vi "Autonomous Independent.vi"() -> ()   [LabVIEW 2015]
doc: "This VI is called when autonomous begins, and will automatically be terminated when autonomous ends. You can carry out timed or sensor driven robot movement independently without needing to return to the caller."
uses:
  <vilib>/Rock Robotics/WPI/Utilities/WPI_GetSetVariantRefNum.vi
  <vilib>/Rock Robotics/Network Tables/NT Read String.vi
  <vilib>/Rock Robotics/Network Tables/NT Write Numeric Array.vi
  <vilib>/Rock Robotics/Network Tables/NT Write Number.vi
  <vilib>/addons/control/pid/pid.llb/PID (DBL).vi
  Robot Global Data.vi
  <vilib>/Rock Robotics/Network Tables/NT Read Number.vi
  <vilib>/addons/control/pid/NI_PID_pid.lvlib
  navX Library v2/navX Library v2.lvlib
panel:
  in  "Aiming Gains":T1={"proportional gain (Kc)"=1.0, "integral time (Ti, min)"=0.01, "derivative time (Td, min)"=0.0} {"derivative time (Td, min)" format="%.3f"; "integral time (Ti, min)" format="%.3f"; "proportional gain (Kc)" format="%.3f"}
  out "Yaw":dbl(graph)
  in  "Target Angle":dbl=30.0
  out "E1 Rate":dbl
  out "E2 Rate":dbl
  out "Yaw Display":dbl
  in  "Single Turn Gains":T1={"proportional gain (Kc)"=0.12, "integral time (Ti, min)"=0.0, "derivative time (Td, min)"=0.0} {"derivative time (Td, min)" format="%.3f"; "integral time (Ti, min)" format="%.3f"; "proportional gain (Kc)" format="%.3f"}
  in  "Yaw":T1={"proportional gain (Kc)"=0.2, "integral time (Ti, min)"=0.0, "derivative time (Td, min)"=0.0} {"derivative time (Td, min)" format="%.3f"; "integral time (Ti, min)" format="%.3f"; "proportional gain (Kc)" format="%.3f"}
  out "Right Motor Speed":dbl(graph)
  out "Left Motor Speed":dbl(graph)
  out "Right Motor":dbl(graph)
  out "Left Motor":dbl(graph)
  in  "Distance":dbl=120.0
  in  "Speed Gains":T1={"proportional gain (Kc)"=0.65, "integral time (Ti, min)"=0.001, "derivative time (Td, min)"=0.001} {"derivative time (Td, min)" format="%.3f"; "integral time (Ti, min)" format="%.3f"; "proportional gain (Kc)" format="%.3f"}
  out "E2 Dist":dbl
  out "E1 Dist":dbl
  # "Be sure to right-click and choose Data Operations>>Make Current Value default if you want to save the array values with the VI"
  # "Encoder Distance Traveled"
  # "Speed we are assigning the motors and Encoder Rate"
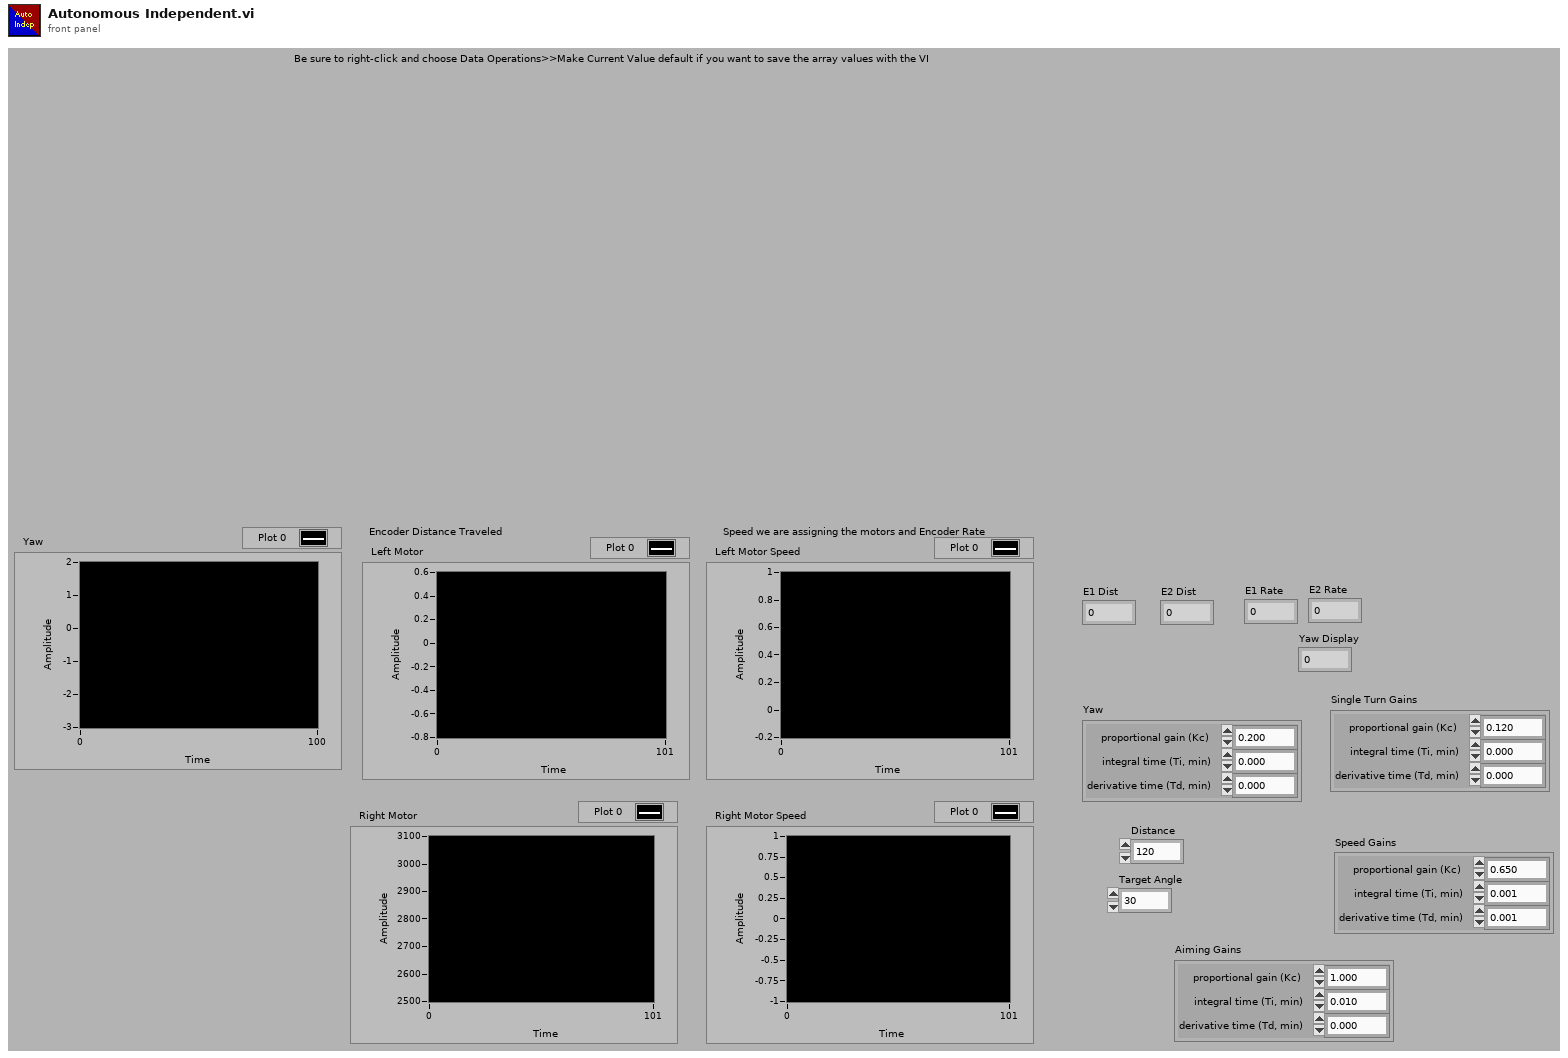
[diagram p1: front panel]
types:
  T1 = cluster{"proportional gain (Kc)":dbl, "integral time (Ti, min)":dbl, "derivative time (Td, min)":dbl}
  T2 = typedef "WPI_JoystickDevRef.ctl" = cluster{"Device":T3}
  T3 = typedef "WPI_JoystickDeviceEnum.ctl" = enum16{"USB 0", "USB 1", "USB 2", "USB 3", "USB 4", "USB 5"}
  T4 = typedef "navX Library v2.lvlib/Z900_navX_DeviceTypeDef.ctl" = cluster{"Interface":cluster{"Protocol":T5, "Update Rate (4Hz-60Hz)":u8, "navX Open TypeDef":variant}, "Notify Packet":refnum<notifier>, "Loop VI Refnum":refnum<vi>, "Ready to Close Occurrence Refnum":refnum<k4>}
  T5 = typedef "navX Library v2.lvlib/Z900_navX_ProtocolTypeDef.ctl" = enum16{"SERIAL", "I2C", "SPI"}
  T6 = typedef "WPI_EncoderDevRef.ctl" = cluster{"DevStatus":errorcluster, "EncoderIndex":T7, "CounterIndex":T8, "DistancePerCount":dbl, "Decoding Type":T9}
  T7 = typedef "FPGA_EncoderIdx.ctl" = enum8{"Enc 0", "Enc 1", "Enc 2", "Enc 3", "Enc 4", "Enc 5", "Enc 6", "Enc 7", "Invalid"}
  T8 = typedef "FPGA_CounterCtrSystemIndex.ctl" = enum8{"Ctr 0", "Ctr 1", "Ctr 2", "Ctr 3", "Ctr 4", "Ctr 5", "Ctr 6", "Ctr 7", "Invalid"}
  T9 = typedef "WPI_EncoderType.ctl" = enum16{"1x", "2x", "4x"}
  T10 = cluster{"Yaw":dbl, "Roll":dbl, "Pitch":dbl, "Heading":dbl, "Fused Heading":dbl}
  T11 = typedef "WPI_RobotDriveDevRef.ctl" = cluster{"DevStatus":errorcluster, "Motors[]":T12[], "Square Inputs":bool, "Max Output":dbl}
  T12 = typedef "WPI_MotorControlDeviceRef.ctl" = cluster{"DeviceStatus":errorcluster, "Type":T13, "PWM":cluster{"PWM Channel":T14, "DeadBand":T15}, "CAN":cluster{"Device Number":u8, "Control Mode":T16, "Semaphore":T17, "Max Vout":dbl, "TalonSRX Control Mode":T18}, "Invert":bool}
  T13 = typedef "WPI_MotorControlType.ctl" = enum16{"PWM", "CAN", "CANTalonSRX"}
  T14 = typedef "FPGA_DIOPWMChannel.ctl" = enum8{"PWM 0", "PWM 1", "PWM 2", "PWM 3", "PWM 4", "PWM 5", "PWM 6", "PWM 7", "PWM 8", "PWM 9", "PWM MXP 0", "PWM MXP 1", "PWM MXP 2", "PWM MXP 3", "PWM MXP 4", "PWM MXP 5", "PWM MXP 6", "PWM MXP 7", "PWM MXP 8", "PWM MXP 9", "Invalid"}
  T15 = typedef "WPI_PWMDeadband.ctl" = cluster{"Name":string, "maxPositivePwm":i32, "minPositivePwm":i32, "centerPwm":i32, "maxNegativePwm":i32, "minNegativePwm":i32, "angularRange":u16}
  T16 = typedef "WPI_CANJaguar_ControlMode.ctl" = enum8{"Percent VBus", "Current", "Speed", "Position", "Voltage"}
  T17 = typedef "Semaphore RefNum" = refnum<k1>
  T18 = typedef "WPI_CANTalonSRX_APIControlMode.ctl" = enum8{"Percent VBus", "Speed", "Position", "Slave", "Unchanged / Invalid", "Voltage Compensation", "Current", "Motion Profile"}
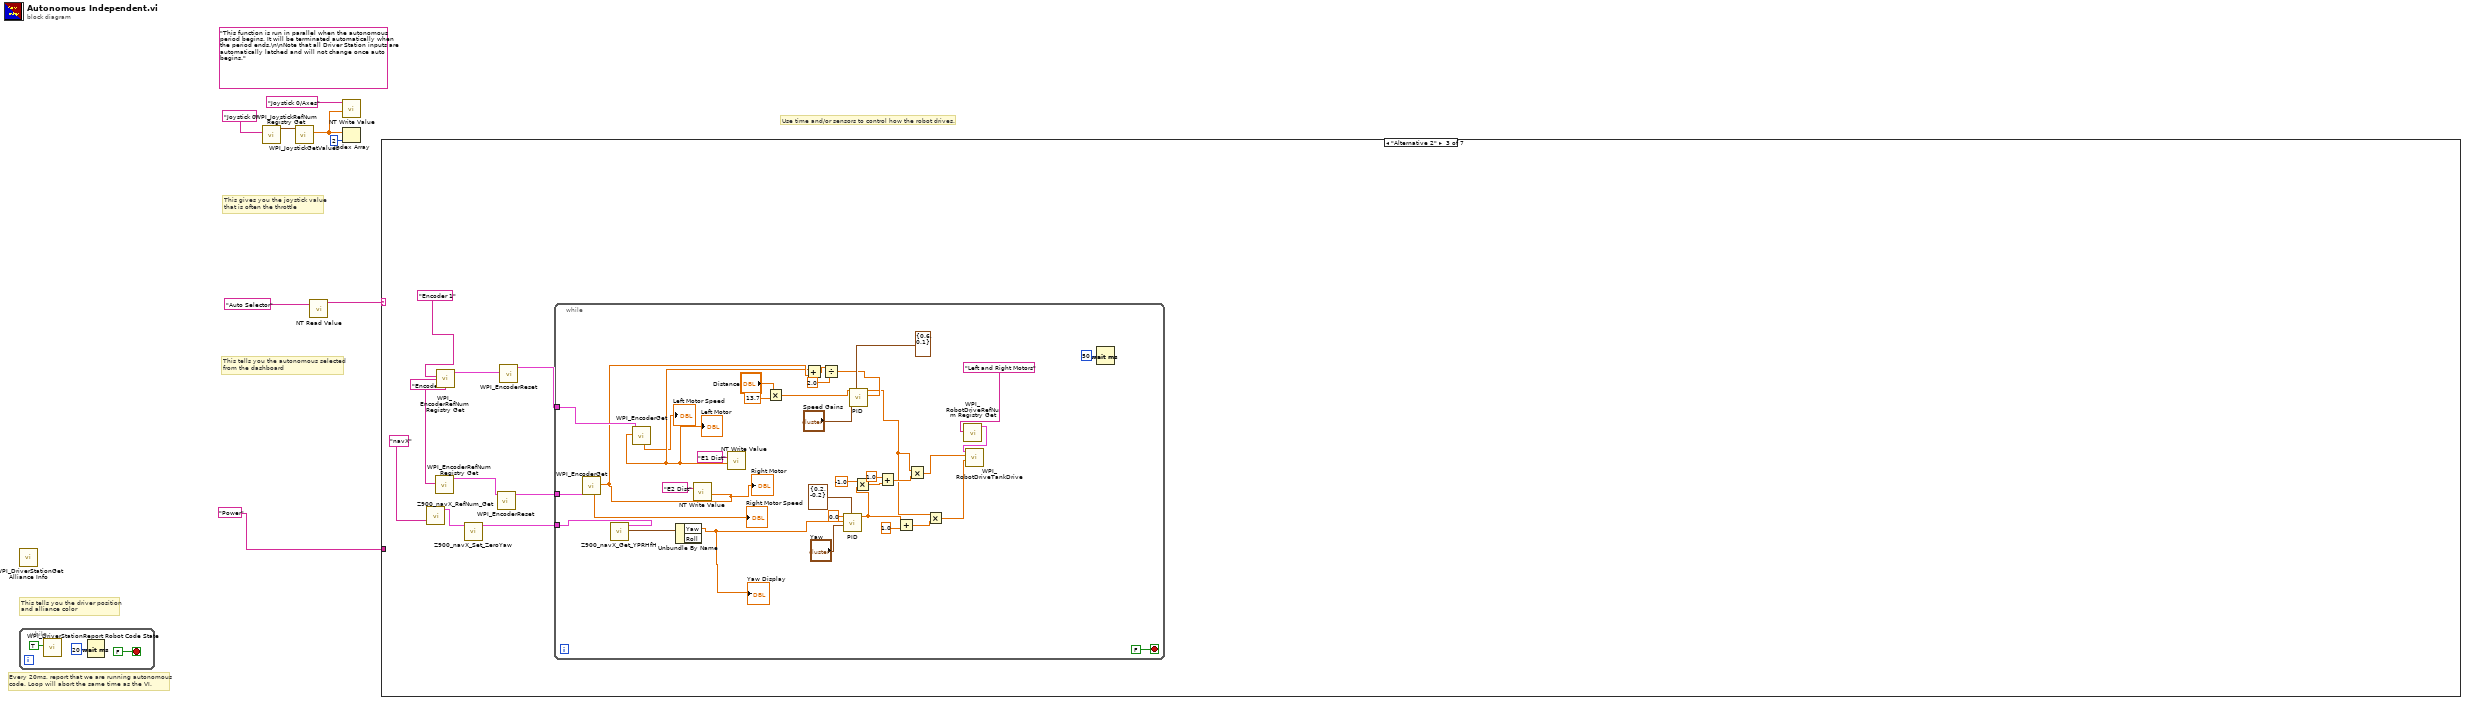
[diagram p0: block diagram]
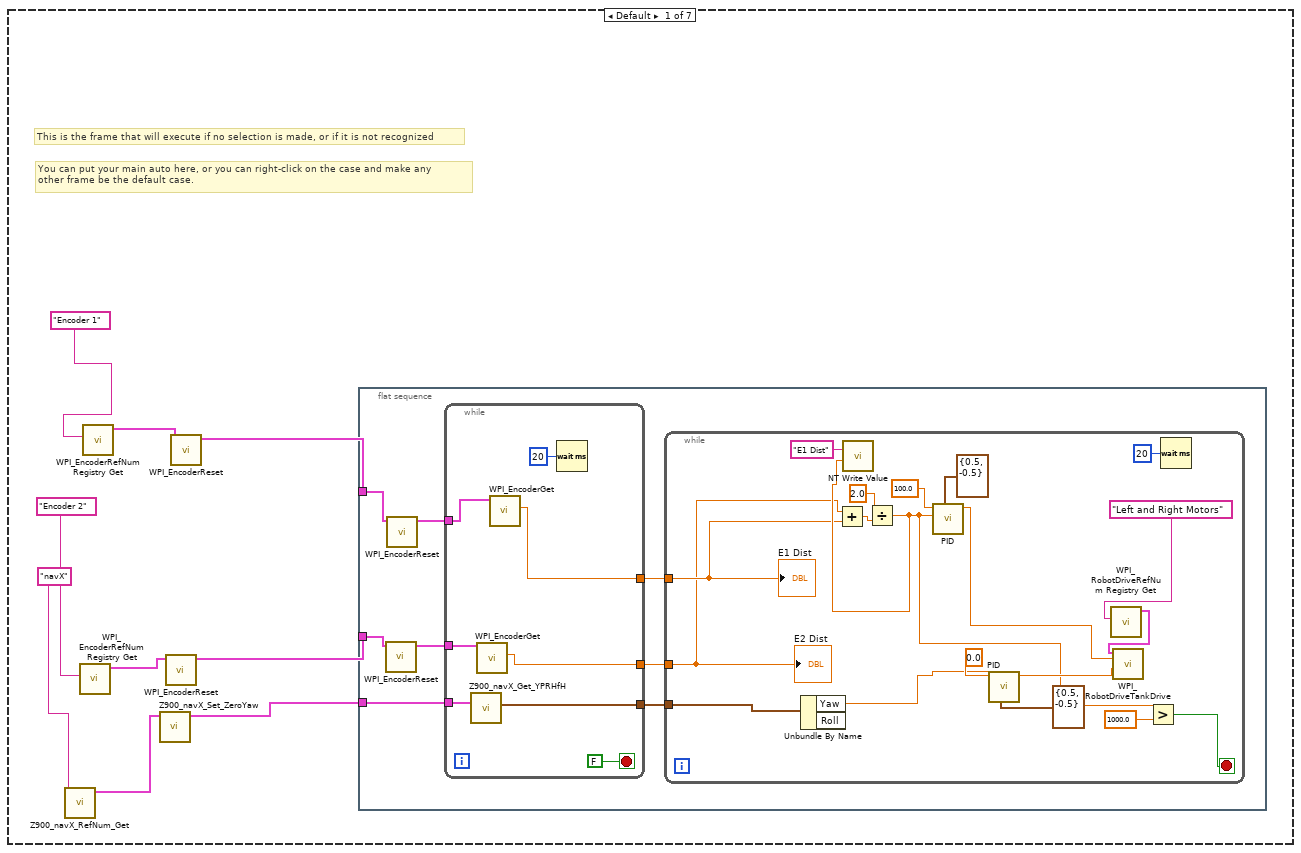
[diagram p2: hidden frame]
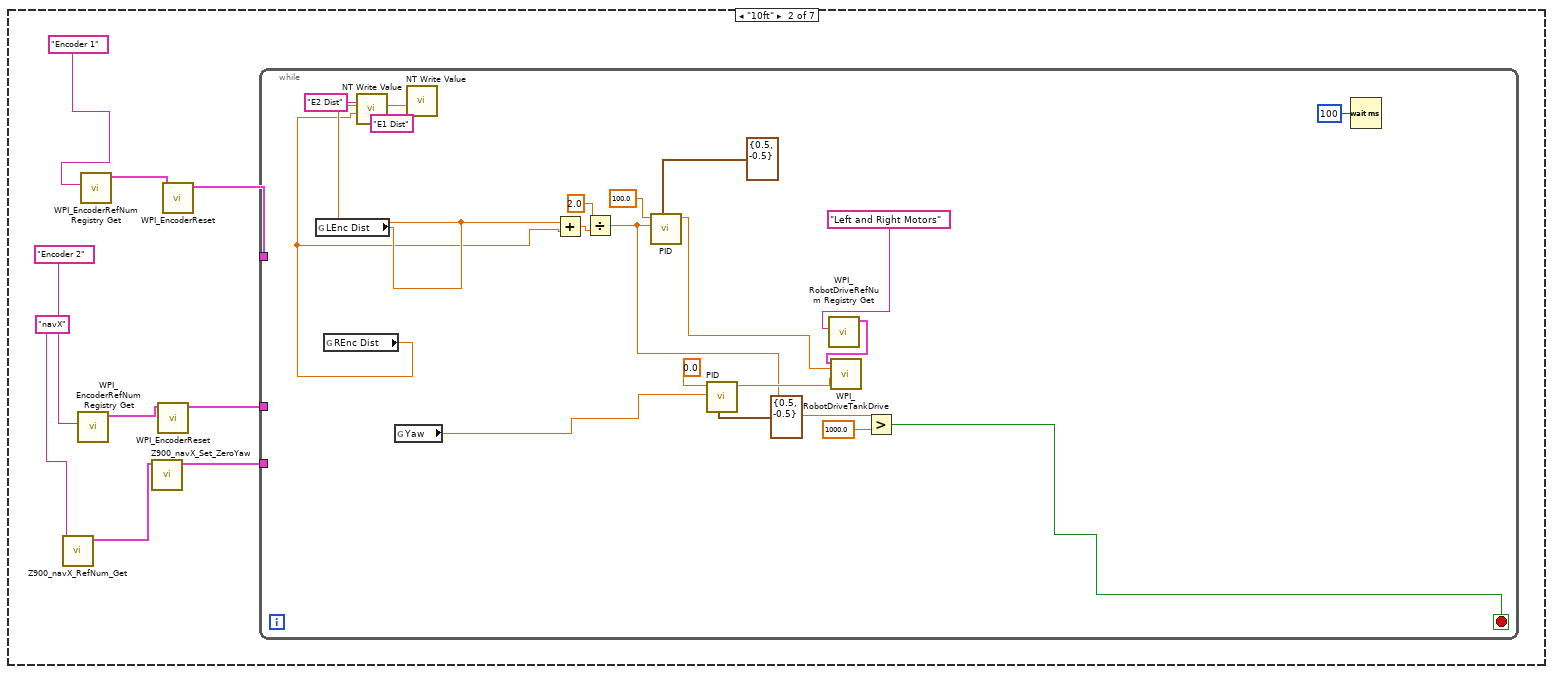
[diagram p3: hidden frame]
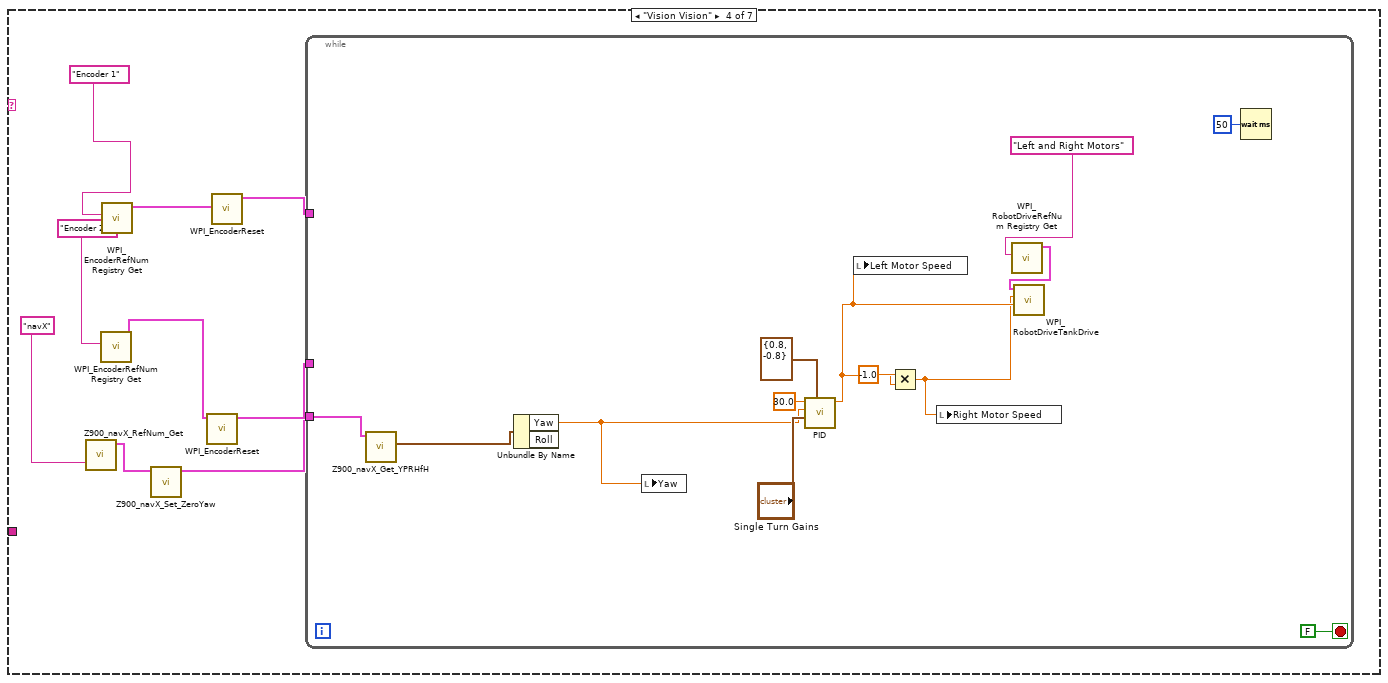
[diagram p4: hidden frame]
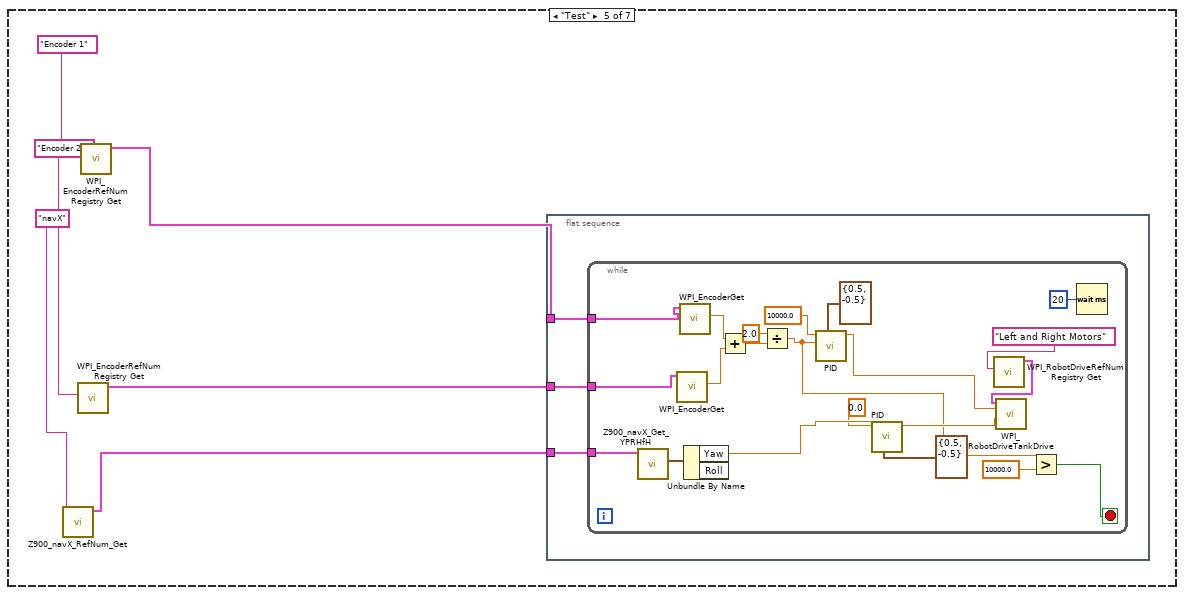
[diagram p5: hidden frame]
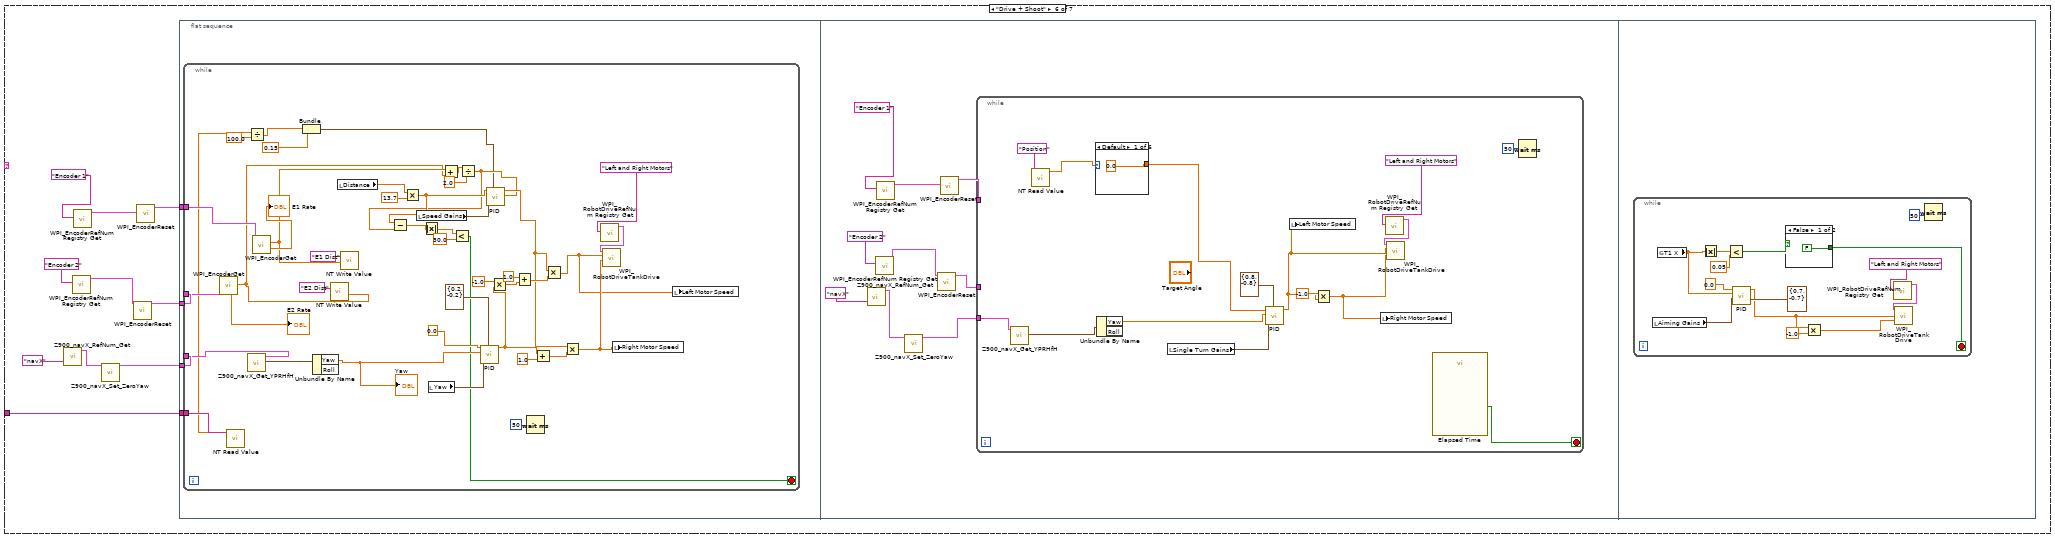
[diagram p6: hidden frame]
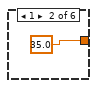
[diagram p7: hidden frame]
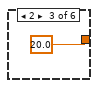
[diagram p8: hidden frame]
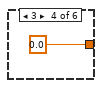
[diagram p9: hidden frame]
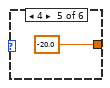
[diagram p10: hidden frame]
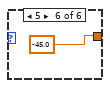
[diagram p11: hidden frame]
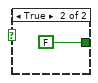
[diagram p12: hidden frame]
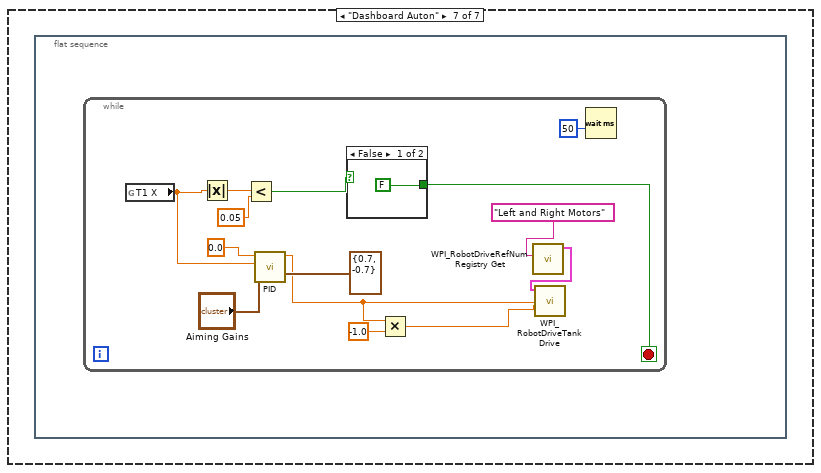
[diagram p13: hidden frame]
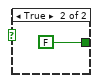
[diagram p14: hidden frame]
diagram:
  (unwired) "This function is run in parallel when the autonomous period begins. It will be terminated automatically when the period ends.\n\nNote that all Driver Station inputs are automatically latched and will not change once auto begins."
  # "This tells you the autonomous selected\nfrom the dashboard"
  # "Every 20ms, report that we are running autonomous\ncode. Loop will abort the same time as the VI."
  # "This gives you the joystick value\nthat is often the throttle"
  # "Use time and/or sensors to control how the robot drives."
  # "This tells you the driver position\nand alliance color"
  n1 = while {
    stop <- FALSE stop-if-true
    n2 = call <vilib>:"WPI_DriverStationReport Robot Code State.vi"("Autonomous"=TRUE) -> ()  [unwired: 10 in, 1 out]
    n3 = Wait (ms)(milliseconds to wait=u32 20) -> ()  [unwired: 1 out]
  }
  n4 = call <vilib>:"WPI_DriverStationGet Alliance Info.vi"() -> ()  [unwired: 12 out]
  n5 = call <vilib>:"WPI_JoystickRefNum Registry Get.vi"("refnum name"="Joystick 0") -> ("JoystickDevRef"=w7:T2)  [unwired: 1 in, 9 out]
  n6 = call <vilib>:"WPI_JoystickGetValues.vi"("JoystickDevRef"=w7) -> ("Axes"=w3:dbl[])  [unwired: 6 in, 4 out]
  n7 = call-poly <vilib>:"NT Read Value.vi"("Name"="Auto Selector") -> ("String"=w4:string)  [unwired: 9 in, 1 out]
  n8 = call-poly <vilib>:"NT Write Value.vi"("Numeric Array"=w3, "Name"="Joystick 0/Axes") -> ()  [unwired: 9 in, 1 out]
  n9 = Index Array(array=w3, index=2) -> ()  [unwired: 1 out]
  n10 = case shown="\"Alternative 2\"" w4 {
    tunnel: "Power" ("Name") -> [_ _ _ _ _ w181 _]
    frame Default {
      # "You can put your main auto here, or you can right-click on the case and make any\nother frame be the default case."
      # "This is the frame that will execute if no selection is made, or if it is not recognized"
      n11 = call "Z900_navX_RefNum_Get.vi"("refnum name"="navX") -> ("navX Device"=w14:T4)  [unwired: 9 in, 1 out]
      n12 = call <vilib>:"WPI_EncoderRefNum Registry Get.vi"("refnum name"="Encoder 2") -> ("EncoderDevRef"=w16:T6)  [unwired: 9 in, 1 out]
      n13 = call <vilib>:"WPI_EncoderRefNum Registry Get.vi"("refnum name"="Encoder 1") -> ("EncoderDevRef"=w18:T6)  [unwired: 9 in, 1 out]
      n14 = call "Z900_navX_Set_ZeroYaw.vi"("navX Device"=w14) -> ("navX Device"=w13:T4)  [unwired: 9 in, 1 out]
      n15 = call <vilib>:"WPI_EncoderReset.vi"("EncoderDevRef"=w16) -> ("EncoderDevRef"=w15:T6)  [unwired: 9 in, 1 out]
      n16 = call <vilib>:"WPI_EncoderReset.vi"("EncoderDevRef"=w18) -> ("EncoderDevRef"=w17:T6)  [unwired: 9 in, 1 out]
      n17 = flat-sequence {
        tunnel: w17 -> [w28]
        tunnel: w15 -> [w27]
        tunnel: w13 -> [w26]
        frame #0 {
          n18 = call <vilib>:"WPI_EncoderReset.vi"("EncoderDevRef"=w27) -> ("EncoderDevRef"=w25:T6)  [unwired: 9 in, 1 out]
          n19 = call <vilib>:"WPI_EncoderReset.vi"("EncoderDevRef"=w28) -> ("EncoderDevRef"=w24:T6)  [unwired: 9 in, 1 out]
          n20 = while {
            tunnel: w26 -> [w33]
            tunnel: w25 -> [w34]
            tunnel: w24 -> [w35]
            tunnel: [w32] -> w23
            tunnel: [w31] -> w22
            tunnel: [w30] -> w21
            stop <- FALSE stop-if-true
            n21 = call "Z900_navX_Get_YPRHfH.vi"("navX Device"=w33) -> ("YRPHfH"=w32:T10)  [unwired: 7 in, 3 out]
            n22 = call <vilib>:"WPI_EncoderGet.vi"("EncoderDevRef"=w34) -> ("Distance"=w31:dbl)  [unwired: 5 in, 5 out]
            n23 = call <vilib>:"WPI_EncoderGet.vi"("EncoderDevRef"=w35) -> ("Distance"=w30:dbl)  [unwired: 5 in, 5 out]
            n24 = Wait (ms)(milliseconds to wait=u32 20) -> ()  [unwired: 1 out]
          }
          n25 = while {
            tunnel: w23 -> [w40]
            tunnel: w22 -> [w38]
            tunnel: w21 -> [w39]
            stop <- w44 stop-if-true
            n26 = Unbundle By Name(w40) -> ("Yaw"=w41:dbl)  [unwired: 1 out]
            n27 = Add(x=w38, y=w39) -> (x+y=w55:dbl)
            n28 = Divide(x=2.0, y=w55) -> (x/y=w43:dbl)
            n29 = call-poly <vilib>:"NT Write Value.vi"("Numeric"=w43, "Name"="E1 Dist") -> ()  [unwired: 9 in, 1 out]
            n30 = call-poly <vilib>:"PID.vi"("output range"=cluster{"output high":dbl, "output low":dbl} {"output high"=0.5, "output low"=-0.5}, "process variable"=w43, "setpoint"=100.0) -> ("output"=w48:dbl)  [unwired: 7 in, 1 out]
            n31 = call-poly <vilib>:"PID.vi"("output range"=cluster{"output high":dbl, "output low":dbl} {"output high"=0.5, "output low"=-0.5}, "process variable"=w41, "setpoint"=0.0) -> ("output"=w47:dbl)  [unwired: 7 in, 1 out]
            n32 = call <vilib>:"WPI_RobotDriveRefNum Registry Get.vi"("refnum name"="Left and Right Motors") -> ("RobotDriveDevRef"=w50:T11)  [unwired: 9 in, 1 out]
            n33 = call <vilib>:"WPI_RobotDriveTankDrive.vi"("Right axis value"=w47, "Left axis value"=w48, "RobotDriveDevRef"=w50) -> ()  [unwired: 6 in, 3 out]
            n34 = Greater?(x=w43, y=1000.0) -> (0:w44:bool)
            n35 = Wait (ms)(milliseconds to wait=u32 20) -> ()  [unwired: 1 out]
            "E2 Dist" <- w38
            "E1 Dist" <- w39
          }
        }
      }
    }
    frame "10ft" {
      n36 = call "Z900_navX_RefNum_Get.vi"("refnum name"="navX") -> ("navX Device"=w58:T4)  [unwired: 9 in, 1 out]
      n37 = call <vilib>:"WPI_EncoderRefNum Registry Get.vi"("refnum name"="Encoder 2") -> ("EncoderDevRef"=w60:T6)  [unwired: 9 in, 1 out]
      n38 = call <vilib>:"WPI_EncoderRefNum Registry Get.vi"("refnum name"="Encoder 1") -> ("EncoderDevRef"=w62:T6)  [unwired: 9 in, 1 out]
      n39 = call "Z900_navX_Set_ZeroYaw.vi"("navX Device"=w58) -> ("navX Device"=w57:T4)  [unwired: 9 in, 1 out]
      n40 = call <vilib>:"WPI_EncoderReset.vi"("EncoderDevRef"=w60) -> ("EncoderDevRef"=w59:T6)  [unwired: 9 in, 1 out]
      n41 = call <vilib>:"WPI_EncoderReset.vi"("EncoderDevRef"=w62) -> ("EncoderDevRef"=w61:T6)  [unwired: 9 in, 1 out]
      n42 = while {
        tunnel: w61 -> [_]
        tunnel: w59 -> [_]
        tunnel: w57 -> [_]
        stop <- w65 stop-if-true
        n43 = global read "Robot Global Data.vi" "LEnc Dist"() -> (w68:dbl)
        n44 = global read "Robot Global Data.vi" "REnc Dist"() -> (w67:dbl)
        n45 = call-poly <vilib>:"NT Write Value.vi"("Numeric"=w67, "Name"="E2 Dist") -> ()  [unwired: 9 in, 1 out]
        n46 = global read "Robot Global Data.vi" "Yaw"() -> (w66:dbl)
        n47 = call-poly <vilib>:"NT Write Value.vi"("Numeric"=w68, "Name"="E1 Dist") -> ()  [unwired: 9 in, 1 out]
        n48 = Add(x=w68, y=w67) -> (x+y=w82:dbl)
        n49 = Divide(x=2.0, y=w82) -> (x/y=w72:dbl)
        n50 = call-poly <vilib>:"PID.vi"("output range"=cluster{"output high":dbl, "output low":dbl} {"output high"=0.5, "output low"=-0.5}, "process variable"=w72, "setpoint"=100.0) -> ("output"=w76:dbl)  [unwired: 7 in, 1 out]
        n51 = call-poly <vilib>:"PID.vi"("output range"=cluster{"output high":dbl, "output low":dbl} {"output high"=0.5, "output low"=-0.5}, "process variable"=w66, "setpoint"=0.0) -> ("output"=w75:dbl)  [unwired: 7 in, 1 out]
        n52 = call <vilib>:"WPI_RobotDriveRefNum Registry Get.vi"("refnum name"="Left and Right Motors") -> ("RobotDriveDevRef"=w78:T11)  [unwired: 9 in, 1 out]
        n53 = call <vilib>:"WPI_RobotDriveTankDrive.vi"("Right axis value"=w75, "Left axis value"=w76, "RobotDriveDevRef"=w78) -> ()  [unwired: 6 in, 3 out]
        n54 = Greater?(x=w72, y=1000.0) -> (0:w65:bool)
        n55 = Wait (ms)(milliseconds to wait=u32 100) -> ()  [unwired: 1 out]
      }
    }
    frame "Alternative 2" {
      n56 = call "Z900_navX_RefNum_Get.vi"("refnum name"="navX") -> ("navX Device"=w85:T4)  [unwired: 9 in, 1 out]
      n57 = call <vilib>:"WPI_EncoderRefNum Registry Get.vi"("refnum name"="Encoder 2") -> ("EncoderDevRef"=w87:T6)  [unwired: 9 in, 1 out]
      n58 = call <vilib>:"WPI_EncoderRefNum Registry Get.vi"("refnum name"="Encoder 1") -> ("EncoderDevRef"=w89:T6)  [unwired: 9 in, 1 out]
      n59 = call "Z900_navX_Set_ZeroYaw.vi"("navX Device"=w85) -> ("navX Device"=w84:T4)  [unwired: 9 in, 1 out]
      n60 = call <vilib>:"WPI_EncoderReset.vi"("EncoderDevRef"=w87) -> ("EncoderDevRef"=w86:T6)  [unwired: 9 in, 1 out]
      n61 = call <vilib>:"WPI_EncoderReset.vi"("EncoderDevRef"=w89) -> ("EncoderDevRef"=w88:T6)  [unwired: 9 in, 1 out]
      n62 = while {
        tunnel: w88 -> [w121]
        tunnel: w86 -> [w120]
        tunnel: w84 -> [w119]
        stop <- FALSE stop-if-true
        n63 = call <vilib>:"WPI_EncoderGet.vi"("EncoderDevRef"=w120) -> ("Distance"=w110:dbl, "Rate"=→"Right Motor Speed":dbl)  [unwired: 5 in, 4 out]
        "Right Motor" <- w110
        n64 = call "Z900_navX_Get_YPRHfH.vi"("navX Device"=w119) -> ("YRPHfH"=w122:T10)  [unwired: 7 in, 3 out]
        n65 = call <vilib>:"WPI_EncoderGet.vi"("EncoderDevRef"=w121) -> ("Distance"=w109:dbl, "Rate"=→"Left Motor Speed":dbl)  [unwired: 5 in, 4 out]
        "Left Motor" <- w109
        n66 = Unbundle By Name(w122) -> ("Yaw"=w95:dbl)  [unwired: 1 out]
        "Yaw Display" <- w95
        n67 = call-poly <vilib>:"NT Write Value.vi"("Numeric"=w110, "Name"="E2 Dist") -> ()  [unwired: 9 in, 1 out]
        n68 = call-poly <vilib>:"NT Write Value.vi"("Numeric"=w109, "Name"="E1 Dist") -> ()  [unwired: 9 in, 1 out]
        n69 = Multiply(x="Distance", y=13.7) -> (x*y=w111:dbl)
        n70 = Add(x=w109, y=w110) -> (x+y=w116:dbl)
        n71 = Divide(x=w116, y=2.0) -> (x/y=w114:dbl)
        n72 = call-poly <vilib>:"PID.vi"("output range"=cluster{"output high":dbl, "output low":dbl} {"output high"=0.2, "output low"=-0.2}, "PID gains"="Yaw", "process variable"=w95, "setpoint"=0.0) -> ("output"=w99:dbl)  [unwired: 6 in, 1 out]
        n73 = call-poly <vilib>:"PID.vi"("output range"=cluster{"output high":dbl, "output low":dbl} {"output high"=0.6, "output low"=0.1}, "PID gains"="Speed Gains", "process variable"=w114, "setpoint"=w111) -> ("output"=w96:dbl)  [unwired: 6 in, 1 out]
        n74 = Multiply(x=-1.0, y=w99) -> (x*y=w100:dbl)
        n75 = Add(x=1.0, y=w100) -> (x+y=w101:dbl)
        n76 = Add(x=w99, y=1.0) -> (x+y=w102:dbl)
        n77 = Multiply(x=w96, y=w101) -> (x*y=w93:dbl)
        n78 = Multiply(x=w96, y=w102) -> (x*y=w94:dbl)
        n79 = call <vilib>:"WPI_RobotDriveRefNum Registry Get.vi"("refnum name"="Left and Right Motors") -> ("RobotDriveDevRef"=w124:T11)  [unwired: 9 in, 1 out]
        n80 = call <vilib>:"WPI_RobotDriveTankDrive.vi"("Right axis value"=w94, "Left axis value"=w93, "RobotDriveDevRef"=w124) -> ()  [unwired: 6 in, 3 out]
        n81 = Wait (ms)(milliseconds to wait=u32 50) -> ()  [unwired: 1 out]
      }
    }
    frame "Vision Vision" {
      n82 = call "Z900_navX_RefNum_Get.vi"("refnum name"="navX") -> ("navX Device"=w130:T4)  [unwired: 9 in, 1 out]
      n83 = call <vilib>:"WPI_EncoderRefNum Registry Get.vi"("refnum name"="Encoder 2") -> ("EncoderDevRef"=w132:T6)  [unwired: 9 in, 1 out]
      n84 = call <vilib>:"WPI_EncoderRefNum Registry Get.vi"("refnum name"="Encoder 1") -> ("EncoderDevRef"=w134:T6)  [unwired: 9 in, 1 out]
      n85 = call "Z900_navX_Set_ZeroYaw.vi"("navX Device"=w130) -> ("navX Device"=w129:T4)  [unwired: 9 in, 1 out]
      n86 = call <vilib>:"WPI_EncoderReset.vi"("EncoderDevRef"=w132) -> ("EncoderDevRef"=w131:T6)  [unwired: 9 in, 1 out]
      n87 = call <vilib>:"WPI_EncoderReset.vi"("EncoderDevRef"=w134) -> ("EncoderDevRef"=w133:T6)  [unwired: 9 in, 1 out]
      n88 = while {
        tunnel: w133 -> [_]
        tunnel: w131 -> [_]
        tunnel: w129 -> [w144]
        stop <- FALSE stop-if-true
        n89 = call "Z900_navX_Get_YPRHfH.vi"("navX Device"=w144) -> ("YRPHfH"=w143:T10)  [unwired: 7 in, 3 out]
        n90 = Unbundle By Name(w143) -> ("Yaw"=w138:dbl)  [unwired: 1 out]
        n91 = local write "Yaw"(w138) -> ()
        n92 = call-poly <vilib>:"PID.vi"("output range"=cluster{"output high":dbl, "output low":dbl} {"output high"=0.8, "output low"=-0.8}, "PID gains"="Single Turn Gains", "process variable"=w138, "setpoint"=30.0) -> ("output"=w140:dbl)  [unwired: 6 in, 1 out]
        n93 = local write "Left Motor Speed"(w140) -> ()
        n94 = Multiply(x=-1.0, y=w140) -> (x*y=w139:dbl)
        n95 = local write "Right Motor Speed"(w139) -> ()
        n96 = call <vilib>:"WPI_RobotDriveRefNum Registry Get.vi"("refnum name"="Left and Right Motors") -> ("RobotDriveDevRef"=w149:T11)  [unwired: 9 in, 1 out]
        n97 = call <vilib>:"WPI_RobotDriveTankDrive.vi"("Right axis value"=w140, "Left axis value"=w139, "RobotDriveDevRef"=w149) -> ()  [unwired: 6 in, 3 out]
        n98 = Wait (ms)(milliseconds to wait=u32 50) -> ()  [unwired: 1 out]
      }
    }
    frame "Test" {
      n99 = call "Z900_navX_RefNum_Get.vi"("refnum name"="navX") -> ("navX Device"=w151:T4)  [unwired: 9 in, 1 out]
      n100 = call <vilib>:"WPI_EncoderRefNum Registry Get.vi"("refnum name"="Encoder 2") -> ("EncoderDevRef"=w152:T6)  [unwired: 9 in, 1 out]
      n101 = call <vilib>:"WPI_EncoderRefNum Registry Get.vi"("refnum name"="Encoder 1") -> ("EncoderDevRef"=w153:T6)  [unwired: 9 in, 1 out]
      n102 = flat-sequence {
        tunnel: w153 -> [w159]
        tunnel: w152 -> [w158]
        tunnel: w151 -> [w157]
        frame #0 {
          n103 = while {
            tunnel: w159 -> [w179]
            tunnel: w158 -> [w178]
            tunnel: w157 -> [w169]
            stop <- w160 stop-if-true
            n104 = call "Z900_navX_Get_YPRHfH.vi"("navX Device"=w169) -> ("YRPHfH"=w180:T10)  [unwired: 7 in, 3 out]
            n105 = call <vilib>:"WPI_EncoderGet.vi"("EncoderDevRef"=w178) -> ("Distance"=w175:dbl)  [unwired: 5 in, 5 out]
            n106 = call <vilib>:"WPI_EncoderGet.vi"("EncoderDevRef"=w179) -> ("Distance"=w176:dbl)  [unwired: 5 in, 5 out]
            n107 = Unbundle By Name(w180) -> ("Yaw"=w171:dbl)  [unwired: 1 out]
            n108 = Add(x=w176, y=w175) -> (x+y=w174:dbl)
            n109 = Divide(x=2.0, y=w174) -> (x/y=w162:dbl)
            n110 = call-poly <vilib>:"PID.vi"("output range"=cluster{"output high":dbl, "output low":dbl} {"output high"=0.5, "output low"=-0.5}, "process variable"=w162, "setpoint"=10000.0) -> ("output"=w165:dbl)  [unwired: 7 in, 1 out]
            n111 = call-poly <vilib>:"PID.vi"("output range"=cluster{"output high":dbl, "output low":dbl} {"output high"=0.5, "output low"=-0.5}, "process variable"=w171, "setpoint"=0.0) -> ("output"=w164:dbl)  [unwired: 7 in, 1 out]
            n112 = call <vilib>:"WPI_RobotDriveRefNum Registry Get.vi"("refnum name"="Left and Right Motors") -> ("RobotDriveDevRef"=w167:T11)  [unwired: 9 in, 1 out]
            n113 = call <vilib>:"WPI_RobotDriveTankDrive.vi"("Right axis value"=w164, "Left axis value"=w165, "RobotDriveDevRef"=w167) -> ()  [unwired: 6 in, 3 out]
            n114 = Greater?(x=w162, y=10000.0) -> (0:w160:bool)
            n115 = Wait (ms)(milliseconds to wait=u32 20) -> ()  [unwired: 1 out]
          }
        }
      }
    }
    frame "Drive + Shoot" {
      n116 = call "Z900_navX_RefNum_Get.vi"("refnum name"="navX") -> ("navX Device"=w189:T4)  [unwired: 9 in, 1 out]
      n117 = call <vilib>:"WPI_EncoderRefNum Registry Get.vi"("refnum name"="Encoder 2") -> ("EncoderDevRef"=w187:T6)  [unwired: 9 in, 1 out]
      n118 = call <vilib>:"WPI_EncoderRefNum Registry Get.vi"("refnum name"="Encoder 1") -> ("EncoderDevRef"=w185:T6)  [unwired: 9 in, 1 out]
      n119 = call "Z900_navX_Set_ZeroYaw.vi"("navX Device"=w189) -> ("navX Device"=w190:T4)  [unwired: 9 in, 1 out]
      n120 = call <vilib>:"WPI_EncoderReset.vi"("EncoderDevRef"=w187) -> ("EncoderDevRef"=w188:T6)  [unwired: 9 in, 1 out]
      n121 = call <vilib>:"WPI_EncoderReset.vi"("EncoderDevRef"=w185) -> ("EncoderDevRef"=w186:T6)  [unwired: 9 in, 1 out]
      n122 = flat-sequence {
        tunnel: w190 -> [w194]
        tunnel: w188 -> [w193]
        tunnel: w186 -> [w192]
        tunnel: w181 -> [w191]
        frame #0 {
          n123 = while {
            tunnel: w192 -> [w232]
            tunnel: w193 -> [w231]
            tunnel: w194 -> [w230]
            tunnel: w191 -> [w200]
            stop <- w201 stop-if-true
            n124 = call <vilib>:"WPI_EncoderGet.vi"("EncoderDevRef"=w231) -> ("Distance"=w207:dbl, "Rate"=→"E2 Rate":dbl)  [unwired: 5 in, 4 out]
            n125 = call-poly <vilib>:"NT Read Value.vi"("Name"=w200) -> ("Numeric"=w199:dbl)  [unwired: 9 in, 1 out]
            n126 = call "Z900_navX_Get_YPRHfH.vi"("navX Device"=w230) -> ("YRPHfH"=w233:T10)  [unwired: 7 in, 3 out]
            n127 = Divide(x=w199, y=100.0) -> (x/y=w197:dbl)
            n128 = call <vilib>:"WPI_EncoderGet.vi"("EncoderDevRef"=w232) -> ("Distance"=w208:dbl, "Rate"=→"E1 Rate":dbl)  [unwired: 5 in, 4 out]
            n129 = Bundle(w197, "output low"=0.15) -> (w195:cluster{dbl, "output low":dbl})  [unwired: 1 in]
            n130 = Unbundle By Name(w233) -> ("Yaw"=w209:dbl)  [unwired: 1 out]
            "Yaw" <- w209
            n131 = call-poly <vilib>:"NT Write Value.vi"("Numeric"=w207, "Name"="E2 Dist") -> ()  [unwired: 9 in, 1 out]
            n132 = local read "Distance"() -> (w217:dbl)
            n133 = call-poly <vilib>:"NT Write Value.vi"("Numeric"=w208, "Name"="E1 Dist") -> ()  [unwired: 9 in, 1 out]
            n134 = Multiply(x=w217, y=13.7) -> (x*y=w206:dbl)
            n135 = local read "Speed Gains"() -> (w211:T1)
            n136 = local read "Yaw"() -> (w215:T1)
            n137 = Add(x=w208, y=w207) -> (x+y=w229:dbl)
            n138 = Divide(x=w229, y=2.0) -> (x/y=w205:dbl)
            n139 = Subtract(x=w206, y=w205) -> (x-y=w204:dbl)
            n140 = Absolute Value(x=w204) -> (abs(x)=w203:dbl)
            n141 = Less?(x=w203, y=30.0) -> (x < y?=w201:bool)
            n142 = call-poly <vilib>:"PID.vi"("output range"=cluster{"output high":dbl, "output low":dbl} {"output high"=0.2, "output low"=-0.2}, "PID gains"=w215, "process variable"=w209, "setpoint"=0.0) -> ("output"=w222:dbl)  [unwired: 6 in, 1 out]
            n143 = call-poly <vilib>:"PID.vi"("output range"=w195, "PID gains"=w211, "process variable"=w205, "setpoint"=w206) -> ("output"=w219:dbl)  [unwired: 6 in, 1 out]
            n144 = Multiply(x=-1.0, y=w222) -> (x*y=w223:dbl)
            n145 = Add(x=1.0, y=w223) -> (x+y=w224:dbl)
            n146 = Wait (ms)(milliseconds to wait=u32 50) -> ()  [unwired: 1 out]
            n147 = Add(x=w222, y=1.0) -> (x+y=w225:dbl)
            n148 = Multiply(x=w219, y=w224) -> (x*y=w212:dbl)
            n149 = Multiply(x=w219, y=w225) -> (x*y=w214:dbl)
            n150 = call <vilib>:"WPI_RobotDriveRefNum Registry Get.vi"("refnum name"="Left and Right Motors") -> ("RobotDriveDevRef"=w235:T11)  [unwired: 9 in, 1 out]
            n151 = call <vilib>:"WPI_RobotDriveTankDrive.vi"("Right axis value"=w214, "Left axis value"=w212, "RobotDriveDevRef"=w235) -> ()  [unwired: 6 in, 3 out]
            n152 = local write "Right Motor Speed"(w214) -> ()
            n153 = local write "Left Motor Speed"(w212) -> ()
          }
        }
        frame #1 {
          n154 = call "Z900_navX_RefNum_Get.vi"("refnum name"="navX") -> ("navX Device"=w240:T4)  [unwired: 9 in, 1 out]
          n155 = call <vilib>:"WPI_EncoderRefNum Registry Get.vi"("refnum name"="Encoder 2") -> ("EncoderDevRef"=w242:T6)  [unwired: 9 in, 1 out]
          n156 = call <vilib>:"WPI_EncoderRefNum Registry Get.vi"("refnum name"="Encoder 1") -> ("EncoderDevRef"=w244:T6)  [unwired: 9 in, 1 out]
          n157 = call "Z900_navX_Set_ZeroYaw.vi"("navX Device"=w240) -> ("navX Device"=w239:T4)  [unwired: 9 in, 1 out]
          n158 = call <vilib>:"WPI_EncoderReset.vi"("EncoderDevRef"=w242) -> ("EncoderDevRef"=w241:T6)  [unwired: 9 in, 1 out]
          n159 = call <vilib>:"WPI_EncoderReset.vi"("EncoderDevRef"=w244) -> ("EncoderDevRef"=w243:T6)  [unwired: 9 in, 1 out]
          n160 = while {
            tunnel: w243 -> [_]
            tunnel: w241 -> [_]
            tunnel: w239 -> [w258]
            stop <- w251 stop-if-true
            n161 = call "Z900_navX_Get_YPRHfH.vi"("navX Device"=w258) -> ("YRPHfH"=w257:T10)  [unwired: 7 in, 3 out]
            n162 = call-poly <vilib>:"NT Read Value.vi"("Name"="Position") -> ("Numeric"=w248:dbl)  [unwired: 9 in, 1 out]
            n163 = case shown="Default" w248 {
              tunnel: [0.0 35.0 20.0 0.0 -20.0 -45.0] -> w249
              frame Default {
              }
              frame 1 {
              }
              frame 2 {
              }
              frame 3 {
              }
              frame 4 {
              }
              frame 5 {
              }
            }
            n164 = Unbundle By Name(w257) -> ("Yaw"=w255:dbl)  [unwired: 1 out]
            n165 = local read "Single Turn Gains"() -> (w254:T1)
            n166 = call-poly <vilib>:"PID.vi"("output range"=cluster{"output high":dbl, "output low":dbl} {"output high"=0.8, "output low"=-0.8}, "PID gains"=w254, "process variable"=w255, "setpoint"=w249) -> ("output"=w253:dbl)  [unwired: 6 in, 1 out]
            n167 = local write "Left Motor Speed"(w253) -> ()
            n168 = Multiply(x=-1.0, y=w253) -> (x*y=w252:dbl)
            n169 = local write "Right Motor Speed"(w252) -> ()
            n170 = call <vilib>:"WPI_RobotDriveRefNum Registry Get.vi"("refnum name"="Left and Right Motors") -> ("RobotDriveDevRef"=w261:T11)  [unwired: 9 in, 1 out]
            n171 = call <vilib>:"WPI_RobotDriveTankDrive.vi"("Right axis value"=w253, "Left axis value"=w252, "RobotDriveDevRef"=w261) -> ()  [unwired: 6 in, 3 out]
            n172 = call "Elapsed Time"() -> ("Time has Elapsed"=w251:bool)  [unwired: 12 in, 7 out]
            n173 = Wait (ms)(milliseconds to wait=u32 50) -> ()  [unwired: 1 out]
          }
        }
        frame #2 {
          n174 = while {
            stop <- w279 stop-if-true
            n175 = local read "Aiming Gains"() -> (w269:T1)
            n176 = global read "Robot Global Data.vi" "T1 X"() -> (w277:dbl)
            n177 = Absolute Value(x=w277) -> (abs(x)=w282:dbl)
            n178 = Less?(x=w282, y=0.05) -> (x < y?=w280:bool)
            n179 = call-poly <vilib>:"PID.vi"("output range"=cluster{"output high":dbl, "output low":dbl} {"output high"=0.7, "output low"=-0.7}, "PID gains"=w269, "process variable"=w277, "setpoint"=0.0) -> ("output"=w271:dbl)  [unwired: 6 in, 1 out]
            n180 = case shown="False" w280 {
              tunnel: [FALSE FALSE] -> w279
              frame False {
              }
              frame True {
              }
            }
            n181 = Multiply(x=w271, y=-1.0) -> (x*y=w270:dbl)
            n182 = call <vilib>:"WPI_RobotDriveRefNum Registry Get.vi"("refnum name"="Left and Right Motors") -> ("RobotDriveDevRef"=w273:T11)  [unwired: 9 in, 1 out]
            n183 = call <vilib>:"WPI_RobotDriveTankDrive.vi"("Right axis value"=w270, "Left axis value"=w271, "RobotDriveDevRef"=w273) -> ()  [unwired: 6 in, 3 out]
            n184 = Wait (ms)(milliseconds to wait=u32 50) -> ()  [unwired: 1 out]
          }
        }
      }
    }
    frame "Dashboard Auton" {
      n185 = flat-sequence {
        frame #0 {
          n186 = while {
            stop <- w295 stop-if-true
            n187 = global read "Robot Global Data.vi" "T1 X"() -> (w293:dbl)
            n188 = Absolute Value(x=w293) -> (abs(x)=w298:dbl)
            n189 = Less?(x=w298, y=0.05) -> (x < y?=w296:bool)
            n190 = call-poly <vilib>:"PID.vi"("output range"=cluster{"output high":dbl, "output low":dbl} {"output high"=0.7, "output low"=-0.7}, "PID gains"="Aiming Gains", "process variable"=w293, "setpoint"=0.0) -> ("output"=w286:dbl)  [unwired: 6 in, 1 out]
            n191 = case shown="False" w296 {
              tunnel: [FALSE FALSE] -> w295
              frame False {
              }
              frame True {
              }
            }
            n192 = Multiply(x=w286, y=-1.0) -> (x*y=w285:dbl)
            n193 = call <vilib>:"WPI_RobotDriveRefNum Registry Get.vi"("refnum name"="Left and Right Motors") -> ("RobotDriveDevRef"=w288:T11)  [unwired: 9 in, 1 out]
            n194 = call <vilib>:"WPI_RobotDriveTankDrive.vi"("Right axis value"=w285, "Left axis value"=w286, "RobotDriveDevRef"=w288) -> ()  [unwired: 6 in, 3 out]
            n195 = Wait (ms)(milliseconds to wait=u32 50) -> ()  [unwired: 1 out]
          }
        }
      }
    }
  }
